vi "ReadBin.vi"(8 "error in (no error)":errorcluster, 11 "FaceEncoding file":path) -> (0 "error out":errorcluster, 3 "Array":u8[](array[numeric]))   [LabVIEW 2020]
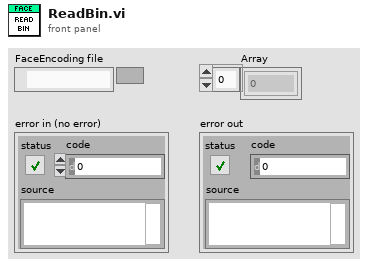
[diagram p1: front panel]
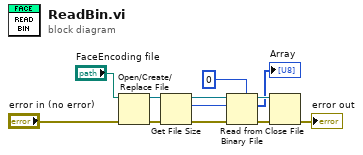
[diagram p0: block diagram]
diagram:
  n1 = Open/Create/Replace File(file path (use dialog)="FaceEncoding file", error in="error in (no error)") -> (refnum out=w7:refnum<file>, error out=w11:errorcluster)  [unwired: 4 in, 1 out]
  n2 = Get File Size(file=w7, error in=w11) -> (refnum out=w10:refnum<file>, size (in bytes)=w8:i64, 0:w9:errorcluster)
  n3 = Read from Binary File(5:u8 0, 8:w9, 10:w8, 11:w10) -> (0:w4:errorcluster, 2:→"Array":u8[], 3:w5:refnum<file>)  [unwired: 2 in, 1 out]
  n4 = Close File(refnum=w5, error in=w4) -> (error out=→"error out":errorcluster)  [unwired: 1 out]
